vi "Lockin Digitizer Signal Recovery.vi"(6 "decimating factor":i32=1, 8 "error in":errorcluster, 9 "Phase in":dbl format="%0.2f", 10 "Frequency":dbl=0.0078125 format="%0.4e", 11 "Input data":dbl[][](array[numeric])) -> (0 "error out":errorcluster, 1 "Phase out":dbl format="%0.2e", 2 "Y":dbl[](array[numeric]), 3 "X":dbl[](array[numeric]))   [LabVIEW 2021]
uses:
  <vilib>/Analysis/NI_AALBase.lvlib
  <vilib>/Analysis/NI_AALPro.lvlib
  <vilib>/Analysis/2dsp.llb/Decimate (single shot, DBL).vi
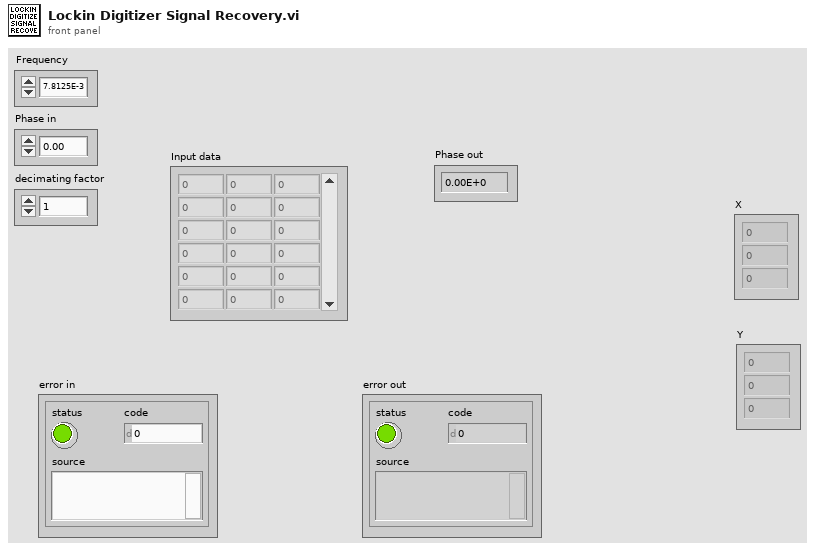
[diagram p1: front panel]
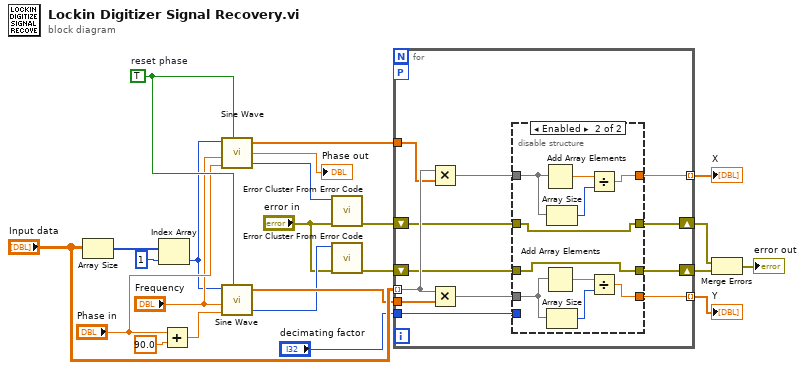
[diagram p0: block diagram]
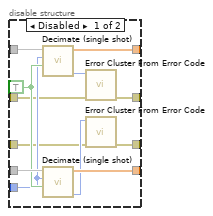
[diagram p2: hidden frame]
diagram:
  w17 = TRUE  # reset phase
  n1 = Array Size(array="Input data") -> (size(s)=w23:i32[])
  n2 = Index Array(array=w23, index=1) -> (element=w12:i32)
  n3 = Add(x="Phase in", y=90.0 ("phase in")) -> (x+y=w14:dbl)
  n4 = call <vilib>:"Sine Wave.vi"("samples"=w12, "frequency"="Frequency", "phase in"="Phase in", "reset phase"=w17) -> ("sine wave"=w18:dbl[], "phase out"=→"Phase out":dbl, "error"=w20:i32)  [unwired: 1 in]
  n5 = call <vilib>:"Sine Wave.vi"("samples"=w12, "frequency"="Frequency", "phase in"=w14, "reset phase"=w17) -> ("sine wave"=w11:dbl[], "error"=w9:i32)  [unwired: 1 in, 1 out]
  n6 = call <vilib>:"Error Cluster From Error Code.vi"("error in (no error)"="error in", "error code (0)"=w20) -> ("error out"=w8:errorcluster)  [unwired: 7 in]
  n7 = call <vilib>:"Error Cluster From Error Code.vi"("error in (no error)"="error in", "error code (0)"=w9) -> ("error out"=w7:errorcluster)  [unwired: 7 in]
  n8 = for {
    tunnel: "Input data" -> [w35] mode=indexing
    tunnel: w18 -> [w34]
    tunnel: w11 -> [w31]
    workers-P: _ -> [_]
    tunnel: "decimating factor" -> [w30]
    tunnel: [w29] -> w4 mode=indexing
    tunnel: [w28] -> w3 mode=indexing
    shift-right: [w26] -> w6
    shift-left: w8 -> [w27]
    shift-right: [w24] -> w5
    shift-left: w7 -> [w25]
    n9 = Multiply(x=w35, y=w34) -> (x*y=w32:dbl[])
    n10 = Multiply(x=w35, y=w31) -> (x*y=w33:dbl[])
    n11 = disable-structure shown="Enabled" {
      disable-tunnel: w33 -> [w47 w51]
      disable-tunnel: w32 -> [w46 w55]
      disable-tunnel: w30 -> [w44 _]
      disable-tunnel: [w43 w54] -> w29
      disable-tunnel: [w42 w50] -> w28
      disable-tunnel: w27 -> [w39 w49]
      disable-tunnel: [w38 w49] -> w26
      disable-tunnel: w25 -> [w37 w48]
      disable-tunnel: [w36 w48] -> w24
      frame Disabled {
        w45 = TRUE ("averaging")
        n12 = call-poly <vilib>:"Decimate (single shot).vi"("averaging"=w45, "decimating factor"=w44, "X"=w46) -> ("error"=w41:i32, "Decimated Array"=w43:dbl[])  [unwired: 7 in]
        n13 = call-poly <vilib>:"Decimate (single shot).vi"("averaging"=w45, "decimating factor"=w44, "X"=w47) -> ("error"=w40:i32, "Decimated Array"=w42:dbl[])  [unwired: 7 in]
        n14 = call <vilib>:"Error Cluster From Error Code.vi"("error in (no error)"=w39, "error code (0)"=w41) -> ("error out"=w38:errorcluster)  [unwired: 7 in]
        n15 = call <vilib>:"Error Cluster From Error Code.vi"("error in (no error)"=w37, "error code (0)"=w40) -> ("error out"=w36:errorcluster)  [unwired: 7 in]
      }
      frame Enabled {
        n16 = Add Array Elements(numeric array=w55) -> (sum=w57:dbl)
        n17 = Add Array Elements(numeric array=w51) -> (sum=w52:dbl)
        n18 = Array Size(array=w55) -> (size(s)=w56:i32)
        n19 = Array Size(array=w51) -> (size(s)=w53:i32)
        n20 = Divide(x=w57, y=w56) -> (x/y=w54:dbl)
        n21 = Divide(x=w52, y=w53) -> (x/y=w50:dbl)
      }
    }
  }
  "Y" <- w3
  "X" <- w4
  n22 = Merge Errors(w6, w5) -> (→"error out":errorcluster)
